vi "XOR4.vi"(2 "B":bool[](array[boolean])=[FALSE, FALSE, FALSE, FALSE, FALSE, FALSE, FALSE, FALSE, FALSE, FALSE, FALSE, FALSE, FALSE, FALSE, FALSE, FALSE], 3 "A":bool[](array[boolean])=[FALSE, FALSE, FALSE, FALSE, FALSE, FALSE, FALSE, FALSE, FALSE, FALSE, FALSE, FALSE, FALSE, FALSE, FALSE, FALSE]) -> (0 "compund equal":bool, 1 "z":bool[](array[boolean]))   [LabVIEW 2012]
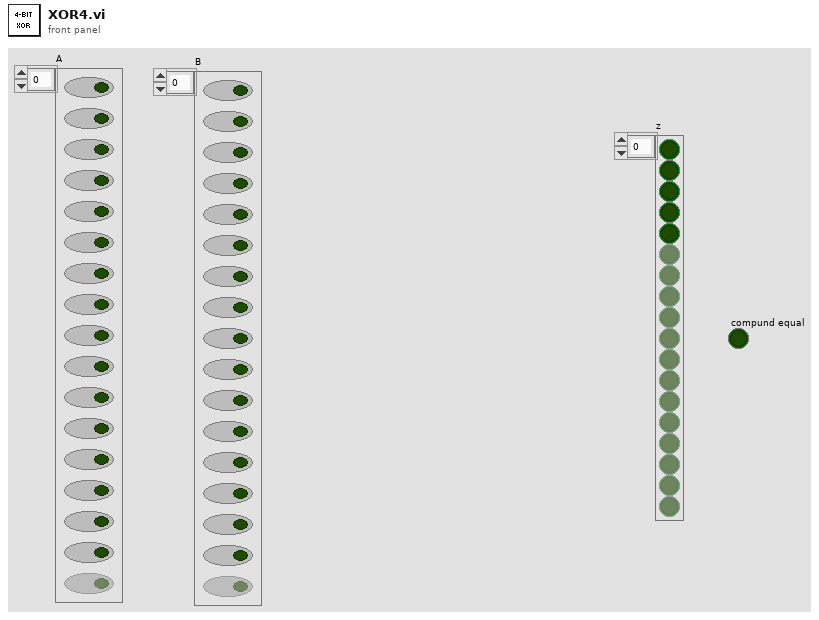
[diagram p1: front panel]
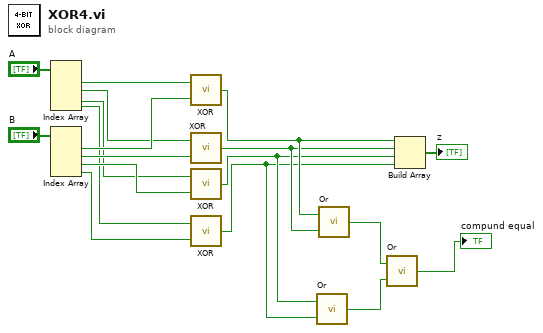
[diagram p0: block diagram]
diagram:
  n1 = Index Array(array="A") -> (element #1=w15:bool, element #2=w14:bool, element #3=w11:bool, element #4=w10:bool)  [unwired: 4 in]
  n2 = Index Array(array="B") -> (element #1=w16:bool, element #2=w13:bool, element #3=w12:bool, element #4=w9:bool)  [unwired: 4 in]
  n3 = call "XOR.vi"("b"=w16, "a"=w15) -> ("x"=w7:bool)
  n4 = call "XOR.vi"("b"=w13, "a"=w14) -> ("x"=w6:bool)
  n5 = call "XOR.vi"("b"=w12, "a"=w11) -> ("x"=w5:bool)
  n6 = call "XOR.vi"("b"=w9, "a"=w10) -> ("x"=w4:bool)
  n7 = call "Or.vi"("b"=w4, "a"=w5) -> ("x"=w2:bool)
  n8 = call "Or.vi"("b"=w6, "a"=w7) -> ("x"=w3:bool)
  n9 = call "Or.vi"("b"=w2, "a"=w3) -> ("x"=→"compund equal":bool)
  n10 = Build Array(w7, w6, w5, w4) -> (→"z":bool[])
